vi "Write FPGA reference.vi"(8 "error in (no error)":errorcluster, 10 "FPGA reference":refnum<k20>, 11 "9770 API in":refnum<class "9770 API.lvclass">) -> (0 "error out":errorcluster, 3 "9770 API out":refnum<class "9770 API.lvclass">)   [LabVIEW 2017, in "9770 API.lvclass"]
uses:
  <vilib>/addons/InsightCM/Devices/Shared/Emsa/Emsa9770API/9770 API.lvclass
  <vilib>/addons/InsightCM/Devices/Shared/Emsa/Emsa9770API/controls/FPGATypeDef.ctl
  <vilib>/addons/InsightCM/Devices/Shared/Emsa/Emsa9770API/9770 API.lvclass/9770 API.ctl
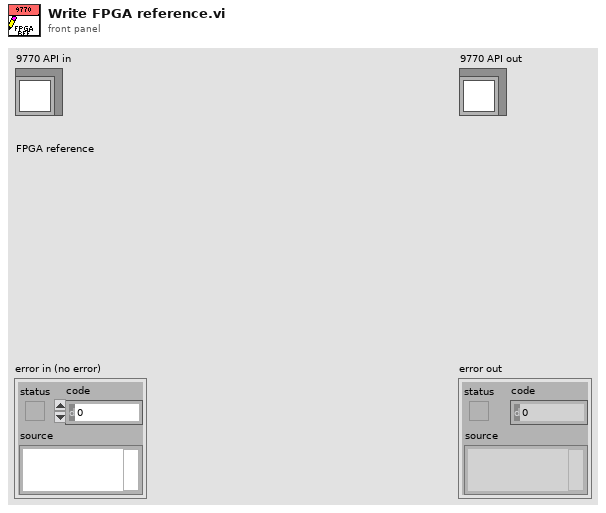
[diagram p1: front panel]
types:
  T1 = typedef "9770 API.lvclass/FPGATypeDef.ctl" = refnum<k20>
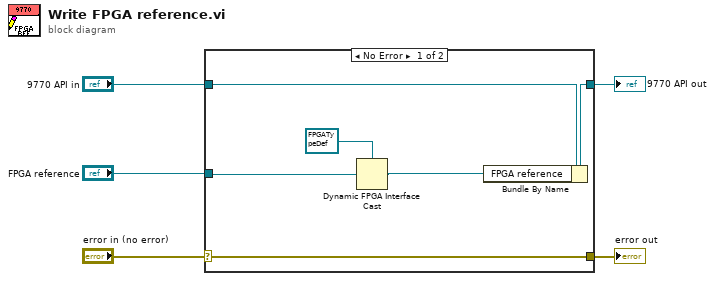
[diagram p0: block diagram]
diagram:
  n1 = case shown="No Error" "error in (no error)" {
    selector: "error in (no error)" -> [w11 w12]
    tunnel: [w11 w12] -> w4
    tunnel: [w9 w13] -> w2
    tunnel: "9770 API in" -> [w10 w13]
    tunnel: "FPGA reference" -> [w6 _]
    frame No Error {
      n2 = Dynamic FPGA Interface Cast(Session In=T1 refnum ("FPGA reference"), Type=w6) -> (Session Out=w7:T1)
      n3 = Bundle By Name(cluster=w10, "FPGA reference"=w7) -> (w9:refnum<class "9770 API.lvclass">)
    }
    frame Error {
    }
  }
  "error out" <- w4
  "9770 API out" <- w2
